vi "Transfer Calibration To EEPROM.vi"(8 "error in (no error)":errorcluster, 10 "Bias Correction Type (1:Accelerometer Bias Correction)":u16(ring)=1 items=["Both Accelerometer And Gyro Bias Corrections", "Accelerometer Bias Correction", "Gyro Bias Correction"], 11 "VISA resource name":refnum<visa-resource-name>) -> (0 "error out":errorcluster, 3 "VISA resource name out":refnum<visa-resource-name>)   [LabVIEW 2012, in "MicroStrain 3DM-GXx.lvlib"]
doc: "Transfer the selected value(s) (Accelerometer Bias Correction and/or Gyro Bias Correction) to EEPROM. The selected offset(s) will be applied to subsequent device power-ups.\n\nIf this VI is not used to save offset values they will be reset to their previous values on device power up."
uses:
  <instrlib>/MicroStrain 3DM-GXx/MicroStrain 3DM-GXx.lvlib
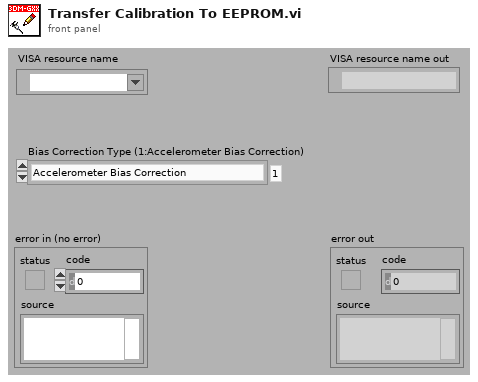
[diagram p1: front panel]
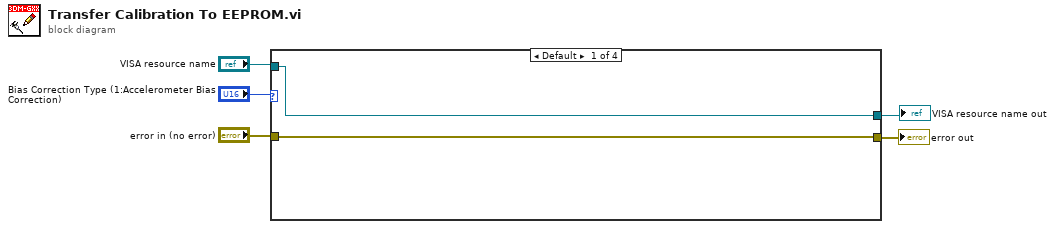
[diagram p0: block diagram]
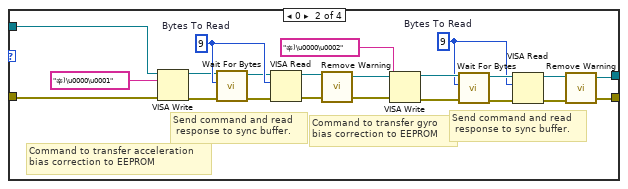
[diagram p2: hidden frame]
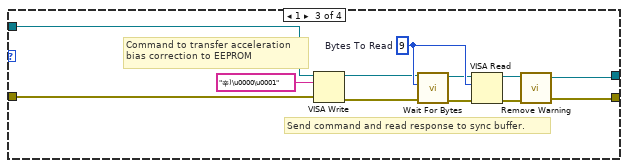
[diagram p3: hidden frame]
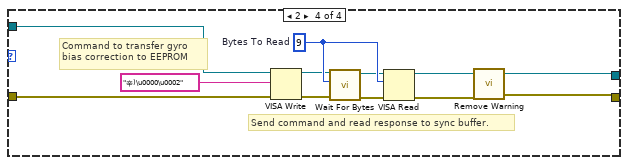
[diagram p4: hidden frame]
diagram:
  n1 = case shown="Default" "Bias Correction Type (1:Accelerometer Bias Correction)" {
    tunnel: "VISA resource name" -> [w7 w17 w34 w47]
    tunnel: "error in (no error)" -> [w6 w16 w35 w46]
    tunnel: [w7 w10 w30 w42] -> w1
    tunnel: [w6 w11 w31 w43] -> w2
    frame Default {
    }
    frame 0 {
      w18 = u32 9  # Bytes To Read
      w29 = u32 9  # Bytes To Read
      # "Send command and read\n response to sync buffer."
      # "Command to transfer gyro \nbias correction to EEPROM"
      # "Send command and read\n response to sync buffer."
      # "Command to transfer acceleration\nbias correction to EEPROM"
      n2 = VISA Write(VISA resource name=w17, write buffer="辛)\u0000\u0001", error in (no error)=w16) -> (VISA resource name out=w25:refnum<visa-resource-name>, error out=w26:errorcluster)  [unwired: 1 out]
      n3 = call <instrlib>:"Wait For Bytes.vi"("error in (no error)"=w26, "Bytes To Read (0)"=w29, "VISA resource name"=w25) -> ("error out"=w27:errorcluster, "VISA resource name out"=w28:refnum<visa-resource-name>)  [unwired: 7 in]
      n4 = VISA Read(VISA resource name=w28, byte count=w29, error in (no error)=w27) -> (VISA resource name out=w15:refnum<visa-resource-name>, error out=w12:errorcluster)  [unwired: 2 out]
      n5 = call <instrlib>:"Remove Warning.vi"("error in (no error)"=w12, "VISA resource name"=w15) -> ("error out"=w13:errorcluster, "VISA resource name out"=w14:refnum<visa-resource-name>)  [unwired: 2 in]
      n6 = VISA Write(VISA resource name=w14, write buffer="辛)\u0000\u0002", error in (no error)=w13) -> (VISA resource name out=w20:refnum<visa-resource-name>, error out=w19:errorcluster)  [unwired: 1 out]
      n7 = call <instrlib>:"Wait For Bytes.vi"("error in (no error)"=w19, "Bytes To Read (0)"=w18, "VISA resource name"=w20) -> ("error out"=w22:errorcluster, "VISA resource name out"=w21:refnum<visa-resource-name>)  [unwired: 7 in]
      n8 = VISA Read(VISA resource name=w21, byte count=w18, error in (no error)=w22) -> (VISA resource name out=w9:refnum<visa-resource-name>, error out=w8:errorcluster)  [unwired: 2 out]
      n9 = call <instrlib>:"Remove Warning.vi"("error in (no error)"=w8, "VISA resource name"=w9) -> ("error out"=w11:errorcluster, "VISA resource name out"=w10:refnum<visa-resource-name>)  [unwired: 2 in]
    }
    frame 1 {
      w41 = u32 9  # Bytes To Read
      # "Send command and read response to sync buffer."
      # "Command to transfer acceleration\nbias correction to EEPROM"
      n10 = VISA Write(VISA resource name=w34, write buffer="辛)\u0000\u0001", error in (no error)=w35) -> (VISA resource name out=w37:refnum<visa-resource-name>, error out=w38:errorcluster)  [unwired: 1 out]
      n11 = call <instrlib>:"Wait For Bytes.vi"("error in (no error)"=w38, "Bytes To Read (0)"=w41, "VISA resource name"=w37) -> ("error out"=w39:errorcluster, "VISA resource name out"=w40:refnum<visa-resource-name>)  [unwired: 7 in]
      n12 = VISA Read(VISA resource name=w40, byte count=w41, error in (no error)=w39) -> (VISA resource name out=w33:refnum<visa-resource-name>, error out=w32:errorcluster)  [unwired: 2 out]
      n13 = call <instrlib>:"Remove Warning.vi"("error in (no error)"=w32, "VISA resource name"=w33) -> ("error out"=w31:errorcluster, "VISA resource name out"=w30:refnum<visa-resource-name>)  [unwired: 2 in]
    }
    frame 2 {
      w53 = u32 9  # Bytes To Read
      # "Send command and read response to sync buffer."
      # "Command to transfer gyro\nbias correction to EEPROM"
      n14 = VISA Write(VISA resource name=w47, write buffer="辛)\u0000\u0002", error in (no error)=w46) -> (VISA resource name out=w49:refnum<visa-resource-name>, error out=w50:errorcluster)  [unwired: 1 out]
      n15 = call <instrlib>:"Wait For Bytes.vi"("error in (no error)"=w50, "Bytes To Read (0)"=w53, "VISA resource name"=w49) -> ("error out"=w51:errorcluster, "VISA resource name out"=w52:refnum<visa-resource-name>)  [unwired: 7 in]
      n16 = VISA Read(VISA resource name=w52, byte count=w53, error in (no error)=w51) -> (VISA resource name out=w45:refnum<visa-resource-name>, error out=w44:errorcluster)  [unwired: 2 out]
      n17 = call <instrlib>:"Remove Warning.vi"("error in (no error)"=w44, "VISA resource name"=w45) -> ("error out"=w43:errorcluster, "VISA resource name out"=w42:refnum<visa-resource-name>)  [unwired: 2 in]
    }
  }
  "VISA resource name out" <- w1
  "error out" <- w2
